vi "Door-Init.vi"(7 "Door reference":refnum<vi>, 8 "error in (no error)":errorcluster, 10 "OutputRequest event ref":T1, 11 "InputData reference":refnum<vi>) -> (0 "error out":errorcluster, 2 "OutputRequest (dup)":T1, 3 "InputData (dup)":refnum<vi>)   [LabVIEW 2015]
doc: "Initializes a Door object.\n\nInputData reference: create reference from Main VI\nOutputRequest event ref: get this from Rack-Init\nDoor reference: which door to initialize?\n\nThe outputs are just duplicates to make it easier to call a bunch of Device-Init functions."
uses:
  Typedefs/Door.ctl
  Rack/Typedefs/OutputRequest refnum.ctl
  Rack/Typedefs/OutputRequest.ctl
  Rack/Typedefs/InputData cluster.ctl
  Rack/Methods/Port drivers/DigitalInput-DataCluster.ctl
panel:
  # "Duration"
  # "Active hi?"
  # "Open"
  # "Close"
  # "(must be on the same \ndevice as open/close)"
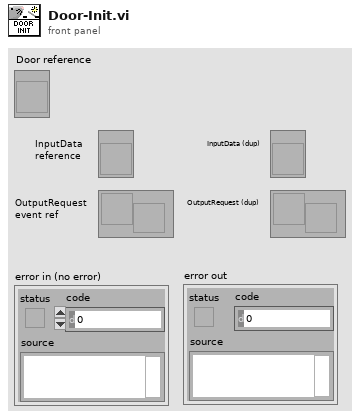
[diagram p1: front panel]
types:
  T1 = typedef "OutputRequest refnum.ctl" = refnum<user-event>
  T2 = typedef "Door.ctl" = cluster{"Open":bool, "Settings":cluster{"Open active hi?":bool, "Open duration":i32, "Close duration":i32, "Close active hi?":bool, "Open portname":string, "Open idx":i32, "Close portname":string, "Close idx":i32, "Timestamp portname":string}, "OutputRequest event ref":T1, "InputData reference":refnum<vi>}
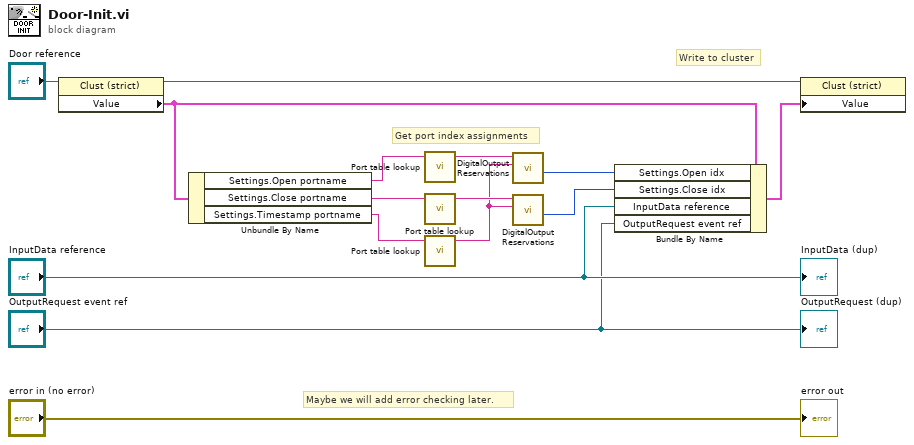
[diagram p0: block diagram]
diagram:
  # "Maybe we will add error checking later."
  # "Write to cluster"
  # "Get port index assignments"
  n1 = property class="Clust (strict)"(reference="Door reference") -> (reference out=w14:refnum<vi>, "Value"=w11:T2)  [unwired: 1 in, 1 out]
  n2 = Unbundle By Name(w11) -> ("Settings.Open portname"=w9:string, "Settings.Close portname"=w7:string, "Settings.Timestamp portname"=w4:string)
  n3 = call "Port table lookup.vi"("Port name"=w9) -> ("Line"=w12:tag)  [unwired: 3 in, 1 out]
  n4 = call "Port table lookup.vi"("Port name"=w7) -> ("Line"=w8:tag)  [unwired: 3 in, 1 out]
  n5 = call "Port table lookup.vi"("Port name"=w4) -> ("Line"=w3:tag)  [unwired: 3 in, 1 out]
  n6 = call "DigitalOutput Reservations.vi"("Timestamp line"=w3, "Line"=w12) -> ("Index assigned"=w10:i32)  [unwired: 2 in, 3 out]
  n7 = call "DigitalOutput Reservations.vi"("Timestamp line"=w3, "Line"=w8) -> ("Index assigned"=w6:i32)  [unwired: 2 in, 3 out]
  n8 = Bundle By Name(cluster=w11, "Settings.Open idx"=w10, "Settings.Close idx"=w6, "InputData reference"="InputData reference", "OutputRequest event ref"="OutputRequest event ref") -> (w13:T2)
  n9 = property class="Clust (strict)"(reference=w14, "Value"=w13) -> ()  [unwired: 1 in, 2 out]
  "error out" <- "error in (no error)"
  "OutputRequest (dup)" <- "OutputRequest event ref"
  "InputData (dup)" <- "InputData reference"
